vi "MyG#G3SubTempl_GetClassAttributes.vi"(0 "reference in":refnum<class "MyG#G3SubTempl.lvclass">, 1 "return data":bool=TRUE, 5 "error in (no error)":errorcluster) -> (14 "reference out":refnum<class "MyG#G3SubTempl.lvclass">, 15 "class attributes ref":T3, 16 "class attributes":T1, 17 "created new":bool, 19 "error out":errorcluster)   [LabVIEW 2020, in "MyG#G3SubTempl.lvclass"]
doc: "Returns a reference and if wanted the actual data values of the class attributes. This method is used by the subclasses to access parent class attributes."
uses:
  MyG#G3SubTempl.lvclass
  ClassAttributesRef.ctl
  protected/ClassAttributes.ctl
  MyG#G3Templ_class/protected/ClassAttributes.ctl
  C:/Program Files (x86)/National Instruments/LabVIEW 2020/vi.lib/addons/_AddQ/G#Object/G#Object.lvclass
  vi.lib/addons/_AddQ/G#Object/G#Object.lvclass
  MyG#G3Templ_class/MyG#G3Templ.lvclass
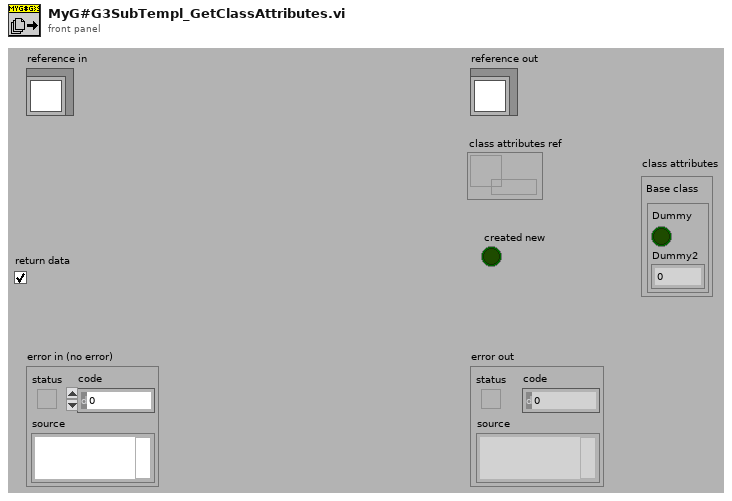
[diagram p1: front panel]
types:
  T1 = typedef "MyG#G3SubTempl.lvclass/ClassAttributes.ctl" = cluster{"Base class":T2}
  T2 = typedef "MyG#G3Templ.lvclass/ClassAttributes.ctl" = cluster{"Dummy":bool, "Dummy2":dbl}
  T3 = typedef "MyG#G3SubTempl.lvclass/ClassAttributesRef.ctl" = refnum<data-value>
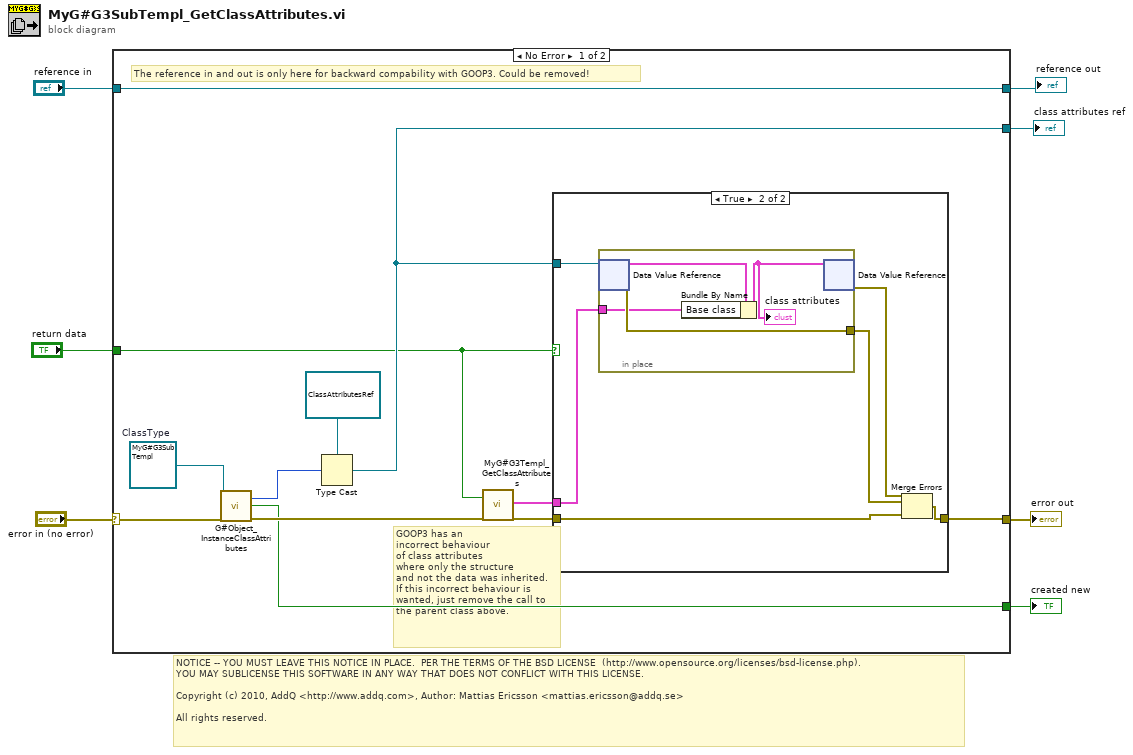
[diagram p0: block diagram]
diagram:
  # "NOTICE -- YOU MUST LEAVE THIS NOTICE IN PLACE.  PER THE TERMS OF THE BSD LICENSE  (http://www.opensource.org/licenses/bsd-license.php).\nYOU MAY SUBLICENSE THIS SOFTWARE IN ANY WAY THAT DOES NOT CONFLICT WITH THIS LICENSE.\n\nCopyright (c) 2010, AddQ <http://www.addq.com>, Author: Mattias Ericsson <mattias.ericsson@addq.se>\n\nAll rights reserved."
  n1 = case shown="No Error" "error in (no error)" {
    selector: "error in (no error)" -> [w12 w32]
    tunnel: [w19 w32] -> w6
    tunnel: [w17 _] -> w5
    tunnel: "return data" -> [w15 _]
    tunnel: [w14 w31] -> w2
    tunnel: "reference in" -> [w14 w31]
    tunnel: [w8 _] -> w1
    frame No Error {
      w10 = refnum<class "MyG#G3SubTempl.lvclass"> refnum  # ClassType
      # "The reference in and out is only here for backward compability with GOOP3. Could be removed!"
      # "GOOP3 has an\nincorrect behaviour\nof class attributes\nwhere only the structure\nand not the data was inherited.\nIf this incorrect behaviour is\nwanted, just remove the call to\nthe parent class above."
      n2 = call "G#Object_InstanceClassAttributes.vi"("reference in"=w10, "error in (no error)"=w12) -> ("static attribute ref"=w9:u32, "created new?"=w8:bool, "error out"=w11:errorcluster)  [unwired: 14 in, 1 out]
      n3 = Type Cast(type=T3 refnum ("data value reference"), x=w9) -> (*(type *) &x=w17:T3)
      n4 = call "MyG#G3Templ_GetClassAttributes.vi"("return data"=w15, "error in (no error)"=w11) -> ("class attributes"=w13:T2, "error out"=w16:errorcluster)  [unwired: 13 in, 3 out]
      n5 = case shown="True" w15 {
        tunnel: w16 -> [w20 w24]
        tunnel: [w20 w25] -> w19
        tunnel: w17 -> [_ w26]
        tunnel: w13 -> [_ w21]
        frame False {
        }
        frame True {
          n6 = in-place {
            in-place-border: [w30] -> w22
            in-place-border: w21 -> [w27]
            n7 = in-place-dvr #1(w26) -> (w29:T1, w30:errorcluster)
            n8 = Bundle By Name(cluster=w29, "Base class"=w27) -> (w28:T1)
            "class attributes" <- w28
            n9 = in-place-dvr #1(w28) -> (w23:errorcluster)  [unwired: 1 out]
          }
          n10 = Merge Errors(w23, w22, w24) -> (w25:errorcluster)
        }
      }
    }
    frame Error {
    }
  }
  "error out" <- w6
  "class attributes ref" <- w5
  "reference out" <- w2
  "created new" <- w1
